vi "year.grid.tester.vi"() -> ()   [LabVIEW 2024]
uses:
  <vilib>/Utility/miscctls.llb/LVBoundsTypeDef.ctl
panel:
  in  "Stop":bool
  in  "offset":cluster{"x":i16, "y":i16}
  in  "pen":T1
  out "Draw Area Size":T2
  in  "end time":timestamp
  in  "start time":timestamp
  out "2D Picture":picture
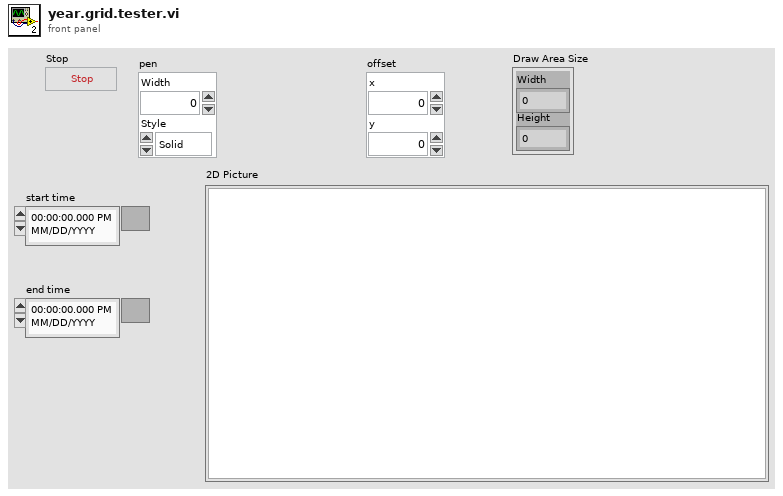
[diagram p1: front panel]
types:
  T1 = cluster{"Width":u16, "Style":enum32{"Solid", "Dash", "Dot", "DashDot", "DashDotDot"}}
  T2 = typedef "LVBoundsTypeDef.ctl" = cluster{"Width":u32, "Height":u32}
  T3 = enum16{"None", "Stacked", "Clockwise", "Counterclockwise"}
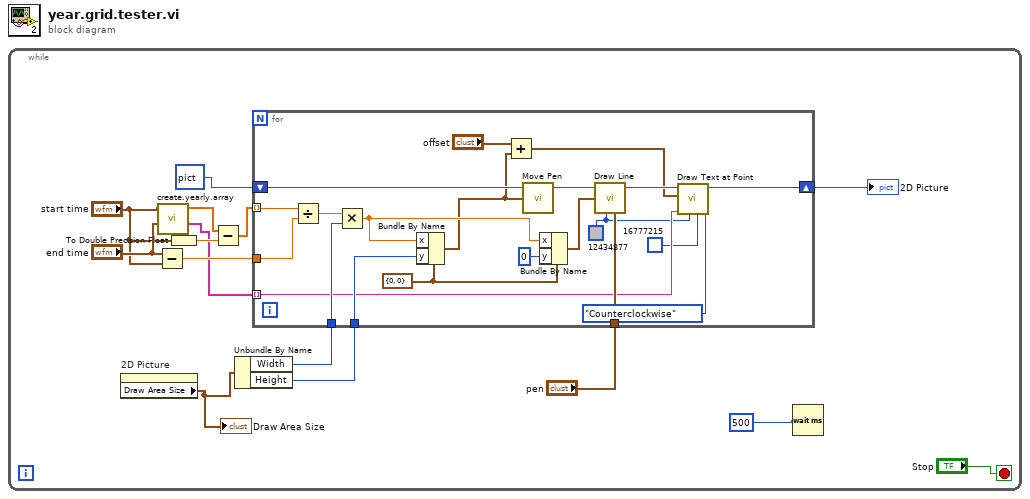
[diagram p0: block diagram]
diagram:
  n1 = while {
    stop <- "Stop" stop-if-true
    n2 = property on="2D Picture" class="Pict"() -> ("Draw Area Size"=w15:T2)  [unwired: 2 in, 2 out]
    "Draw Area Size" <- w15
    n3 = Subtract(x="end time", y="start time") -> (x-y=w13:dbl)
    n4 = call "create.yearly.array.vi"("end time"="end time", "start time"="start time") -> ("names"=w3:string[], "timestamps"=w7:dbl[])  [unwired: 8 in]
    n5 = To Double Precision Float(number="start time") -> (double precision float=w4:dbl)
    n6 = Subtract(x=w7, y=w4) -> (x-y=w5:dbl[])
    n7 = Unbundle By Name(w15) -> ("Width"=w12:u32, "Height"=w9:u32)
    n8 = for {
      tunnel: w5 -> [w36] mode=indexing
      tunnel: w13 -> [w35]
      tunnel: w12 -> [w33]
      shift-right: [w24] -> w10
      shift-left: picture data[5B] ("2D Picture") -> [w32]
      tunnel: w9 -> [w30]
      tunnel: "pen" -> [w26]
      tunnel: w3 -> [w23] mode=indexing
      w19 = u32 12434877 ("color(black)")
      w29 = cluster{"x":i16, "y":i16} {"x"=0, "y"=0} ("new position")
      n9 = Divide(x=w36, y=w35) -> (x/y=w34:dbl)
      n10 = Multiply(x=w34, y=w33) -> (x*y=w28:dbl)
      n11 = Bundle By Name(cluster=w29, "x"=w28, "y"=w30) -> (w17:cluster{"x":i16, "y":i16})
      n12 = Add(x="offset", y=w17) -> (x+y=w16:cluster{"x":i16, "y":i16})
      n13 = call <vilib>:"Move Pen.vi"("new position"=w17, "picture"=w32) -> ("new picture"=w31:picture)  [unwired: 3 in]
      n14 = Bundle By Name(cluster=w29, "x"=w28, "y"=i16 0) -> (w20:cluster{"x":i16, "y":i16})
      n15 = call <vilib>:"Draw Line.vi"("picture"=w31, "end point"=w20, "color(black)"=w19, "pen"=w26) -> ("new picture"=w25:picture)  [unwired: 5 in]
      n16 = call <vilib>:"Draw Text at Point.vi"("text orientation"=T3."Counterclockwise", "BG color(transparent)"=u32 16777215, "text color(black)"=w19, "text"=w23, "origin"=w16, "picture"=w25) -> ("new picture"=w24:picture)  [unwired: 4 in, 1 out]
    }
    "2D Picture" <- w10
    n17 = Wait (ms)(milliseconds to wait=u32 500) -> ()  [unwired: 1 out]
  }
